vi "Begin.vi"(8 "error in":errorcluster) -> (0 "error out":errorcluster)   [LabVIEW 2014]
doc: "Called before other user functions, this VI is expected to open initial I/O refnums, load in file data, and do all program initialization. Notice that the <B>error out</B> terminal is simply used for data flow. Wiring it to other structures or subVIs ensures that this VI runs first."
uses:
  <vilib>/Rock Robotics/WPI/DriverStation/WPI_DriverStationRobotMode2.ctl
  <vilib>/Rock Robotics/WPI/Joystick/WPI_JoystickDeviceEnum.ctl
  <vilib>/Rock Robotics/SystemInterfaces/AI/FPGA_AIGyroChannel.ctl
  <vilib>/Rock Robotics/WPI/Camera/WPI_CameraWhite Balance Values.ctl
  <vilib>/Rock Robotics/WPI/Camera/WPI_CameraExposure Values.ctl
  <vilib>/Rock Robotics/WPI/Solenoid/WPI_SolenoidChannel.ctl
  <vilib>/Rock Robotics/SystemInterfaces/AI/FPGA_AIChannel.ctl
  <vilib>/Rock Robotics/WPI/Accelerometer/ADXL345 Range.ctl
  <vilib>/Rock Robotics/WPI/Accelerometer/WPI_AccelerometerADXL345 Axes.ctl
  <vilib>/Rock Robotics/SystemInterfaces/i2clib/i2c_bus.ctl
  <vilib>/Rock Robotics/SystemInterfaces/DIO/FPGA_DIOChannel.ctl
  <vilib>/Rock Robotics/SystemInterfaces/DIO/FPGA_DIOPWMChannel.ctl
  <vilib>/Rock Robotics/WPI/CAN/TalonSRX/WPI_CANTalonSRX_BrakeOverride.ctl
  Robot Global Data.vi
  <vilib>/Rock Robotics/WPI/RobotDrive/WPI_RobotDriveOpen4MotorWithCANJaguar.vi
  <vilib>/Rock Robotics/WPI/Solenoid/WPI_SolenoidOpenSingle.vi
  <vilib>/Rock Robotics/WPI/Counter/WPI_CounterDigitalInputToDigitalSource.vi
  <vilib>/Rock Robotics/WPI/MotorControl/WPI_MotorControlOpenCANTalonSRX.vi
  <vilib>/Rock Robotics/WPI/Compressor/WPI_CompressorGetSetRefNum.vi
panel:
  out "Discovered Devices":i32[](array[numeric])
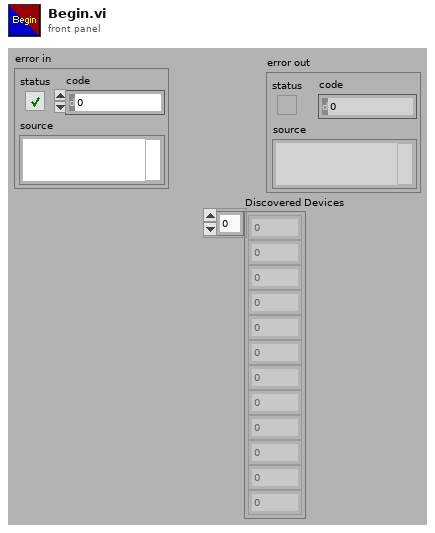
[diagram p1: front panel]
types:
  T1 = typedef "WPI_SolenoidChannel.ctl" = enum8{"Solenoid 0", "Solenoid 1", "Solenoid 2", "Solenoid 3", "Solenoid 4", "Solenoid 5", "Solenoid 6", "Solenoid 7", "Invalid"}
  T2 = typedef "WPI_CANTalonSRX_BrakeOverride.ctl" = enum8{"No Override", "Override to Coast", "Override to Brake"}
  T3 = typedef "FPGA_DIOChannel.ctl" = enum8{"DIO 0", "DIO 1", "DIO 2", "DIO 3", "DIO 4", "DIO 5", "DIO 6", "DIO 7", "DIO 8", "DIO 9", "DIO MXP 0", "DIO MXP 1", "DIO MXP 2", "DIO MXP 3", "DIO MXP 4", "DIO MXP 5", "DIO MXP 6", "DIO MXP 7", "DIO MXP 8", "DIO MXP 9", "DIO MXP 10", "DIO MXP 11", "DIO MXP 12", "DIO MXP 13", "DIO MXP 14", "DIO MXP 15", "Invalid"}
  T4 = typedef "FPGA_DIOPWMChannel.ctl" = enum8{"PWM 0", "PWM 1", "PWM 2", "PWM 3", "PWM 4", "PWM 5", "PWM 6", "PWM 7", "PWM 8", "PWM 9", "PWM MXP 0", "PWM MXP 1", "PWM MXP 2", "PWM MXP 3", "PWM MXP 4", "PWM MXP 5", "PWM MXP 6", "PWM MXP 7", "PWM MXP 8", "PWM MXP 9", "Invalid"}
  T5 = typedef "i2c_bus.ctl" = enum16{"I2C On-Board", "I2C MXP", "Invalid"}
  T6 = typedef "WPI_AccelerometerADXL345 Axes.ctl" = cluster{"X-Axis":bool, "Y-Axis":bool, "Z-Axis":bool}
  T7 = typedef "ADXL345 Range.ctl" = u8
  T8 = typedef "FPGA_AIChannel.ctl" = enum8{"AI 0", "AI 1", "AI 2", "AI 3", "AI MXP 0", "AI MXP 1", "AI MXP 2", "AI MXP 3", "Invalid"}
  T9 = typedef "WPI_CameraExposure Values.ctl" = enum16{"Auto", "Flicker-free 50 Hz", "Flicker-free 60 Hz", "Hold current", "Custom"}
  T10 = typedef "WPI_CameraWhite Balance Values.ctl" = enum16{"Auto", "Fixed indoor", "Fixed outdoor 1", "Fixed outdoor 2", "Fixed fluorescent 1", "Fixed fluorescent 2", "Hold current", "Custom"}
  T11 = typedef "FPGA_AIGyroChannel.ctl" = enum8{"AI 0", "AI 1", "Invalid"}
  T12 = typedef "WPI_JoystickDeviceEnum.ctl" = enum16{"USB 0", "USB 1", "USB 2", "USB 3", "USB 4", "USB 5"}
  T13 = typedef "WPI_DriverStationRobotMode2.ctl" = enum16{"Autonomous Disabled", "Autonomous Enabled", "Teleop Disabled", "Teleop Enabled", "Disconnected", "Finish", "Test Disabled", "Test Enabled", "Emergency Stopped"}
  T14 = typedef "WPI_JoystickDevRef.ctl" = cluster{"Device":T12}
  T15 = typedef "WPI_GyroDevRef.ctl" = cluster{"DevStatus":errorcluster, "Analog Module":T16, "Analog Channel":T8, "Offset":dbl, "Gain (VoltsPerDegree/Second)":dbl}
  T16 = typedef "FPGA_TypedefAnalogModule.ctl" = enum16{"Controller 1"}
  T17 = typedef "WPI_AccelerometerDevRef.ctl" = cluster{"DevStatus":errorcluster, "Controller":T16, "Scaling":T18, "Analog Channels":T19, "I2C Bus":T5, "SPI Bus":T20, "Accel Range":T7, "ADXL345 Axes":T6, "Handle":i32, "Device Address":u8, "Accel Type":enum16{"Analog", "ADXL345 I2C", "ADXL345 SPI", "Internal"}}
  T18 = typedef "WPI_AccelerometerScaling.ctl" = cluster{"Gain (VoltsPerG)":dbl, "Center Voltage":dbl}
  T19 = typedef "WPI_AccelerometerAnalogChannels.ctl" = cluster{"X-Axis":T8, "Y-Axis":T8, "Z-Axis":T8}
  T20 = typedef "spi_bus.ctl" = enum16{"SPI On-Board, CS0", "SPI On-Board, CS1", "SPI On-Board, CS2", "SPI On-Board, CS3", "SPI MXP", "Invalid"}
  T21 = typedef "WPI_RobotDriveDevRef.ctl" = cluster{"DevStatus":errorcluster, "Motors[]":T22[], "Square Inputs":bool, "Max Output":dbl}
  T22 = typedef "WPI_MotorControlDeviceRef.ctl" = cluster{"DeviceStatus":errorcluster, "Type":T23, "PWM":cluster{"Controller":T24, "PWM Channel":T4, "DeadBand":T25}, "CAN":cluster{"Device Number":u8, "Control Mode":T26, "Semaphore":T27, "Max Vout":dbl, "TalonSRX Control Mode":T28}, "Invert":bool, "TransformRef":T29, "InvTransformRef":T29}
  T23 = typedef "WPI_MotorControlType.ctl" = enum16{"PWM", "CAN", "CANTalonSRX"}
  T24 = typedef "FPGA_TypedefDigitalModule.ctl" = enum16{"Controller 1"}
  T25 = typedef "WPI_PWMDeadband.ctl" = cluster{"Name":string, "maxPositivePwm":i32, "minPositivePwm":i32, "centerPwm":i32, "maxNegativePwm":i32, "minNegativePwm":i32, "angularRange":u16}
  T26 = typedef "WPI_CANJaguar_ControlMode.ctl" = enum8{"Percent VBus", "Current", "Speed", "Position", "Voltage"}
  T27 = typedef "Semaphore RefNum" = refnum<k1>
  T28 = typedef "WPI_CANTalonSRX_APIControlMode.ctl" = enum8{"Percent VBus", "Speed", "Position", "Slave", "Unchanged / Invalid"}
  T29 = typedef "WPI_PWMTransform_ConPane.ctl" = refnum<vi>
  T30 = typedef "WPI_SolenoidDevRef.ctl" = cluster{"DevStatus":errorcluster, "Pneumatics Control Module":u8, "Forward Solenoid Channel":T1, "Reverse Solenoid Channel":T1}
  T31 = typedef "WPI_CameraDevRef.ctl" = cluster{"Camera Address":string, "CameraStatus":errorcluster}
  T32 = typedef "WPI_AnalogChannelDevRef.ctl" = cluster{"DevStatus":errorcluster, "Controller":T16, "Analog Channel":T8}
  T33 = typedef "WPI_I2CDevRef.ctl" = cluster{"DevStatus":errorcluster, "Controller":T24, "Device Address":u8, "Handle":i32, "I2C Bus":T5}
  T34 = typedef "WPI_CompressorDevRef.ctl" = cluster{"DevStatus":errorcluster, "Pneumatics Control Module":u8}
  T35 = typedef "WPI_DigitalInputDevRef.ctl" = cluster{"DevStatus":errorcluster, "DIO Channel":T3, "Controller":T24}
  T36 = typedef "WPI_ServoDeviceRef.ctl" = cluster{"DeviceStatus":errorcluster, "Controller":T24, "PWM Channel":T4, "DeadBand":T25}
  T37 = typedef "FPGA_CounterEncoderSourceConvertionLVSourceType.ctl" = cluster{"DevStatus":errorcluster, "AnalogTriggerMode?":bool, "DigitalMode":cluster{"Controller":T24, "DIO Channel":T38}, "AnalogTriggerMode":cluster{"AnalogTriggerIndex":T39, "OutputType":T40}}
  T38 = typedef "FPGA_DIODigitalSourceChannel.ctl" = enum8{"DIO 0", "DIO 1", "DIO 2", "DIO 3", "DIO 4", "DIO 5", "DIO 6", "DIO 7", "DIO 8", "DIO 9", "DIO MXP 0", "DIO MXP 1", "DIO MXP 2", "DIO MXP 3", "DIO MXP 4", "DIO MXP 5", "DIO MXP 6", "DIO MXP 7", "DIO MXP 8", "DIO MXP 9", "DIO MXP 10", "DIO MXP 11", "DIO MXP 12", "DIO MXP 13", "DIO MXP 14", "DIO MXP 15", "Disabled"}
  T39 = typedef "FPGA_AnalogTriggerIndex.ctl" = enum8{"Trig 0", "Trig 1", "Trig 2", "Trig 3", "Trig 4", "Trig 5", "Trig 6", "Trig 7", "Invalid"}
  T40 = typedef "FPGA_AnalogTriggerOutType.ctl" = enum16{"InWindow", "TriggerState", "Rising", "Falling"}
  T41 = typedef "WPI_EncoderDevRef.ctl" = cluster{"DevStatus":errorcluster, "EncoderIndex":T42, "CounterIndex":T43, "DistancePerCount":dbl, "Decoding Type":T44}
  T42 = typedef "FPGA_EncoderIdx.ctl" = enum8{"Enc 0", "Enc 1", "Enc 2", "Enc 3", "Enc 4", "Enc 5", "Enc 6", "Enc 7", "Invalid"}
  T43 = typedef "FPGA_CounterCtrSystemIndex.ctl" = enum8{"Ctr 0", "Ctr 1", "Ctr 2", "Ctr 3", "Ctr 4", "Ctr 5", "Ctr 6", "Ctr 7", "Invalid"}
  T44 = typedef "WPI_EncoderType.ctl" = enum16{"1x", "2x", "4x"}
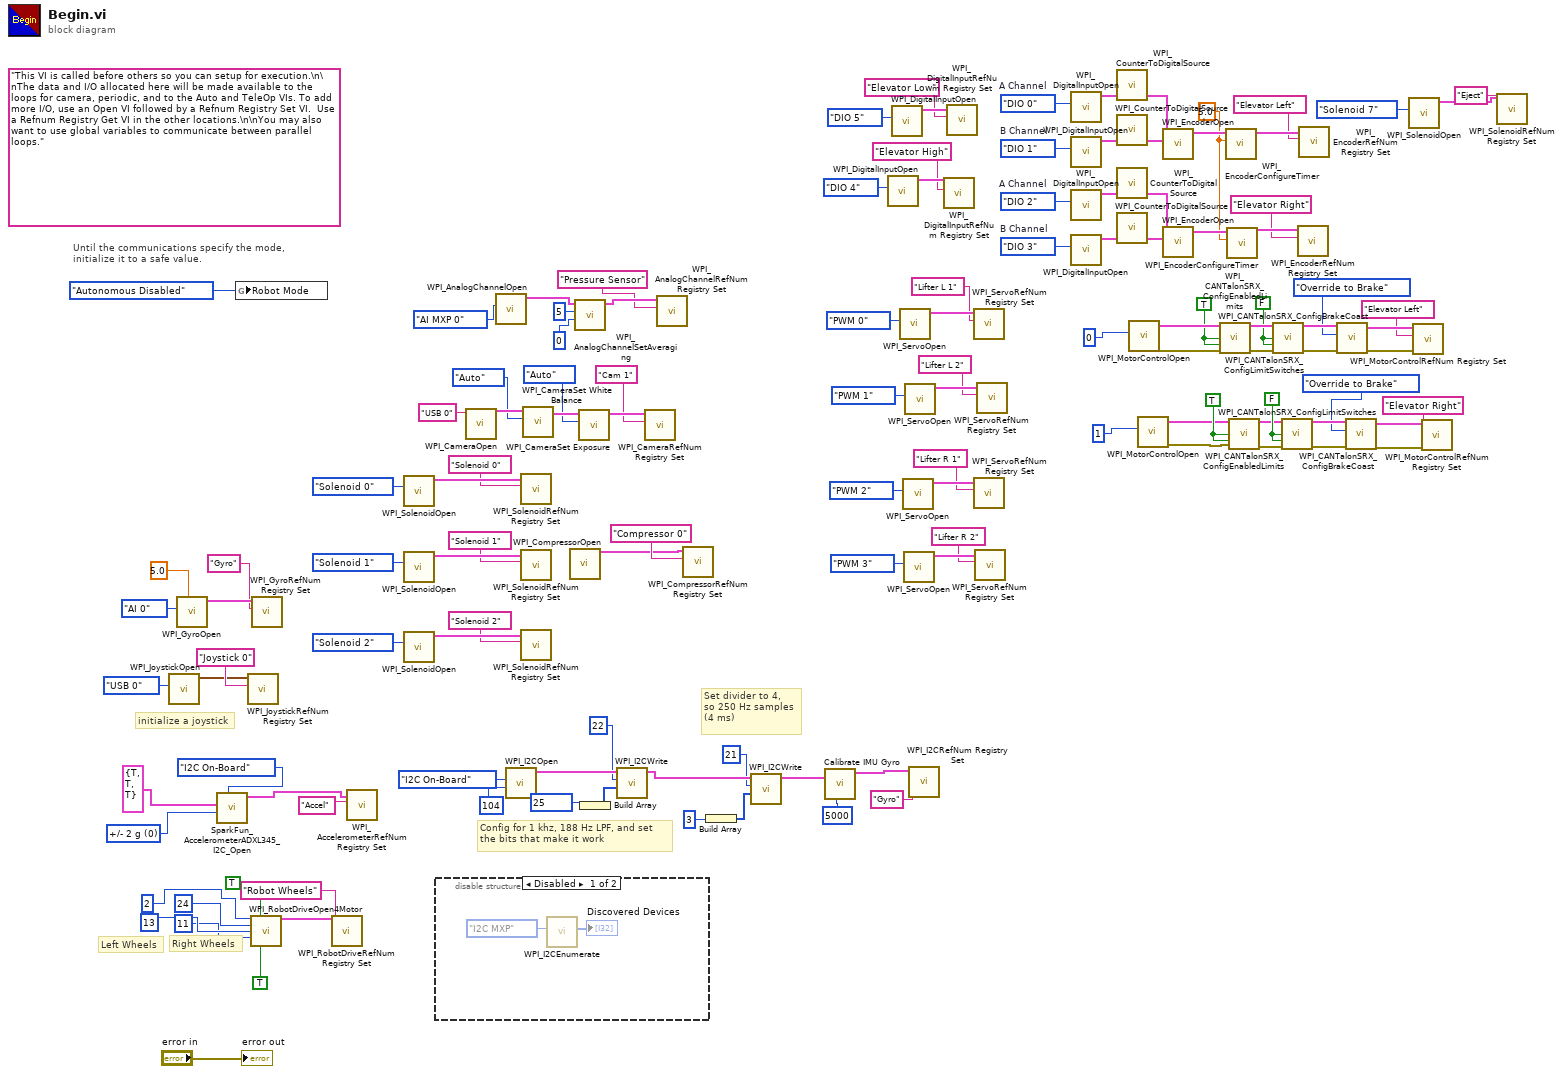
[diagram p0: block diagram]
diagram:
  w17 = FALSE ("Forward Limit Switch Enable")
  w15 = TRUE ("Forward Limit Switch Enable")
  w25 = FALSE ("Forward Limit Switch Enable")
  w27 = TRUE ("Forward Limit Switch Enable")
  w30 = 5.0 ("Minimum Rate")
  w55 = FPGA_DIOChannel."DIO 3"  # B Channel
  w56 = FPGA_DIOChannel."DIO 2"  # A Channel
  w66 = FPGA_DIOChannel."DIO 1"  # B Channel
  w65 = FPGA_DIOChannel."DIO 0"  # A Channel
  w82 = T7 0 items=["+/- 2 g", "+/- 4 g", "+/- 8 g", "+/- 16 g"] ("Accel Range")
  (unwired) "This VI is called before others so you can setup for execution.\n\nThe data and I/O allocated here will be made available to the loops for camera, periodic, and to the Auto and TeleOp VIs. To add more I/O, use an Open VI followed by a Refnum Registry Set VI.  Use a Refnum Registry Get VI in the other locations.\n\nYou may also want to use global variables to communicate between parallel loops."
  # "Set divider to 4, \nso 250 Hz samples\n(4 ms)"
  # "Config for 1 khz, 188 Hz LPF, and set\nthe bits that make it work"
  # "Right Wheels"
  # "Left Wheels"
  # "initialize a joystick"
  # "Until the communications specify the mode,\ninitialize it to a safe value."
  n1 = call <vilib>:"WPI_JoystickOpen.vi"("JoystickDevice"=WPI_JoystickDeviceEnum."USB 0") -> ("JoystickDevRef"=w124:T14)  [unwired: 10 in]
  n2 = call <vilib>:"WPI_GyroOpen.vi"("Calibration Time (s)"=5.0, "Analog Channel"=FPGA_AIGyroChannel."AI 0") -> ("GyroDevRef"=w115:T15)  [unwired: 7 in, 2 out]
  n3 = call "SparkFun_AccelerometerADXL345_I2C_Open.vi"("I2C Bus"=i2c_bus."I2C On-Board", "Accel Range"=w82, "ADXL345 Axes"=T6 {"X-Axis"=TRUE, "Y-Axis"=TRUE, "Z-Axis"=TRUE}) -> ("AccelerometerDevRef"=w84:T17)  [unwired: 7 in, 1 out]
  n4 = global write "Robot Global Data.vi" "Robot Mode"(WPI_DriverStationRobotMode2."Autonomous Disabled" ("Robot Mode")) -> ()
  n5 = call <vilib>:"WPI_JoystickRefNum Registry Set.vi"("refnum name"="Joystick 0", "JoystickDevRef"=w124) -> ()  [unwired: 8 in, 2 out]
  n6 = call-poly <vilib>:"WPI_RobotDriveOpen4Motor.vi"("Rear Left Motor"=u8 2, "Rear Left Motor Inverted"=TRUE, "Rear Right Motor"=u8 24, "Front Left Motor"=u8 13, "Front Right Motor"=u8 11, "Front Left Motor Inverted"=TRUE) -> ("RobotDriveDevRef"=w121:T21)  [unwired: 8 in, 1 out]
  n7 = call <vilib>:"WPI_GyroRefNum Registry Set.vi"("refnum name"="Gyro", "GyroDevRef"=w115) -> ()  [unwired: 8 in, 2 out]
  n8 = call <vilib>:"WPI_RobotDriveRefNum Registry Set.vi"("refnum name"="Robot Wheels", "RobotDriveDevRef"=w121) -> ()  [unwired: 8 in, 2 out]
  n9 = call <vilib>:"WPI_AccelerometerRefNum Registry Set.vi"("refnum name"="Accel", "AccelerometerDevRef"=w84) -> ()  [unwired: 8 in, 2 out]
  n10 = call-poly <vilib>:"WPI_SolenoidOpen.vi"("Solenoid Channel"=WPI_SolenoidChannel."Solenoid 0") -> ("SolenoidDevRef"=w102:T30)  [unwired: 9 in, 1 out]
  n11 = call-poly <vilib>:"WPI_SolenoidOpen.vi"("Solenoid Channel"=WPI_SolenoidChannel."Solenoid 1") -> ("SolenoidDevRef"=w94:T30)  [unwired: 9 in, 1 out]
  n12 = call-poly <vilib>:"WPI_SolenoidOpen.vi"("Solenoid Channel"=WPI_SolenoidChannel."Solenoid 2") -> ("SolenoidDevRef"=w97:T30)  [unwired: 9 in, 1 out]
  n13 = disable-structure shown="Disabled" {
    frame Disabled {
      n14 = call <vilib>:"WPI_I2CEnumerate.vi"("I2C Bus"=i2c_bus."I2C MXP") -> ("Discovered Devices"=→"Discovered Devices":i32[])  [unwired: 10 in]
    }
    frame Enabled {
    }
  }
  n15 = call <vilib>:"WPI_CameraOpen.vi"("Camera Address"="USB 0") -> ("CameraDevRef"=w108:T31)  [unwired: 9 in, 1 out]
  n16 = call <vilib>:"WPI_AnalogChannelOpen.vi"("Analog Channel"=FPGA_AIChannel."AI MXP 0") -> ("AIDeviceRef"=w90:T32)  [unwired: 9 in, 1 out]
  n17 = call <vilib>:"WPI_I2COpen.vi"("Device Address"=104, "I2C Bus"=i2c_bus."I2C On-Board") -> ("I2CDevRef"=w75:T33)  [unwired: 8 in, 1 out]
  n18 = call <vilib>:"WPI_SolenoidRefNum Registry Set.vi"("refnum name"="Solenoid 0", "SolenoidDevRef"=w102) -> ()  [unwired: 8 in, 2 out]
  n19 = call <vilib>:"WPI_SolenoidRefNum Registry Set.vi"("refnum name"="Solenoid 1", "SolenoidDevRef"=w94) -> ()  [unwired: 8 in, 2 out]
  n20 = call <vilib>:"WPI_SolenoidRefNum Registry Set.vi"("refnum name"="Solenoid 2", "SolenoidDevRef"=w97) -> ()  [unwired: 8 in, 2 out]
  n21 = call <vilib>:"WPI_CameraSet White Balance.vi"("White Balance"=WPI_CameraWhite_Balance_Values."Auto", "CameraDevRef"=w108) -> ("CameraDevRef Out"=w106:T31)  [unwired: 8 in, 1 out]
  n22 = call <vilib>:"WPI_CompressorOpen.vi"() -> ("CompressorDevRef"=w98:T34)  [unwired: 14 in, 1 out]
  n23 = call <vilib>:"WPI_AnalogChannelSetAveraging.vi"("OversampleBits"=u8 0, "AverageBits"=u8 5, "AIDeviceRef"=w90) -> ("AIDeviceRef"=w91:T32)  [unwired: 7 in, 1 out]
  n24 = call <vilib>:"WPI_CameraSet Exposure.vi"("Exposure"=WPI_CameraExposure_Values."Auto", "CameraDevRef"=w106) -> ("CameraDevRef Out"=w104:T31)  [unwired: 8 in, 1 out]
  n25 = Build Array(u8 25) -> (w77:u8[])
  n26 = call <vilib>:"WPI_I2CWrite.vi"("I2CDataToSend"=w77, "I2CRegister"=u8 22, "I2CDevRef"=w75) -> ("I2CDevRef"=w78:T33)  [unwired: 7 in, 1 out]
  n27 = call <vilib>:"WPI_CameraRefNum Registry Set.vi"("refnum name"="Cam 1", "CameraDevRef"=w104) -> ()  [unwired: 8 in, 2 out]
  n28 = call <vilib>:"WPI_AnalogChannelRefNum Registry Set.vi"("refnum name"="Pressure Sensor", "AIDeviceRef"=w91) -> ()  [unwired: 8 in, 2 out]
  n29 = call <vilib>:"WPI_CompressorRefNum Registry Set.vi"("refnum name"="Compressor 0", "CompressorDevRef"=w98) -> ()  [unwired: 8 in, 2 out]
  n30 = Build Array(u8 3) -> (w72:u8[])
  n31 = call <vilib>:"WPI_I2CWrite.vi"("I2CDataToSend"=w72, "I2CRegister"=u8 21, "I2CDevRef"=w78) -> ("I2CDevRef"=w79:T33)  [unwired: 7 in, 1 out]
  n32 = call "Calibrate IMU Gyro.vi"("Calib time (ms)"=u32 5000, "I2CDevRef in"=w79) -> ("I2CDevRef out"=w80:T33)  [unwired: 9 in]
  n33 = call <vilib>:"WPI_DigitalInputOpen.vi"("DIO Channel"=FPGA_DIOChannel."DIO 4") -> ("DigitalInputDevRef"=w47:T35)  [unwired: 9 in, 1 out]
  n34 = call <vilib>:"WPI_DigitalInputOpen.vi"("DIO Channel"=FPGA_DIOChannel."DIO 5") -> ("DigitalInputDevRef"=w48:T35)  [unwired: 9 in, 1 out]
  n35 = call <vilib>:"WPI_ServoOpen.vi"("PWM Channel"=FPGA_DIOPWMChannel."PWM 0") -> ("ServoDeviceRef"=w38:T36)  [unwired: 9 in, 1 out]
  n36 = call <vilib>:"WPI_ServoOpen.vi"("PWM Channel"=FPGA_DIOPWMChannel."PWM 2") -> ("ServoDeviceRef"=w36:T36)  [unwired: 9 in, 1 out]
  n37 = call <vilib>:"WPI_ServoOpen.vi"("PWM Channel"=FPGA_DIOPWMChannel."PWM 3") -> ("ServoDeviceRef"=w35:T36)  [unwired: 9 in, 1 out]
  n38 = call <vilib>:"WPI_ServoOpen.vi"("PWM Channel"=FPGA_DIOPWMChannel."PWM 1") -> ("ServoDeviceRef"=w37:T36)  [unwired: 9 in, 1 out]
  n39 = call <vilib>:"WPI_I2CRefNum Registry Set.vi"("refnum name"="Gyro", "I2CDevRef"=w80) -> ()  [unwired: 8 in, 2 out]
  n40 = call <vilib>:"WPI_DigitalInputRefNum Registry Set.vi"("refnum name"="Elevator High", "DigitalInputDevRef"=w47) -> ()  [unwired: 8 in, 2 out]
  n41 = call <vilib>:"WPI_DigitalInputRefNum Registry Set.vi"("refnum name"="Elevator Low", "DigitalInputDevRef"=w48) -> ()  [unwired: 8 in, 2 out]
  n42 = call <vilib>:"WPI_ServoRefNum Registry Set.vi"("refnum name"="Lifter L 1", "ServoDeviceRef"=w38) -> ()  [unwired: 8 in, 2 out]
  n43 = call <vilib>:"WPI_ServoRefNum Registry Set.vi"("refnum name"="Lifter R 1", "ServoDeviceRef"=w36) -> ()  [unwired: 8 in, 2 out]
  n44 = call <vilib>:"WPI_ServoRefNum Registry Set.vi"("refnum name"="Lifter R 2", "ServoDeviceRef"=w35) -> ()  [unwired: 8 in, 2 out]
  n45 = call <vilib>:"WPI_ServoRefNum Registry Set.vi"("refnum name"="Lifter L 2", "ServoDeviceRef"=w37) -> ()  [unwired: 8 in, 2 out]
  n46 = call <vilib>:"WPI_DigitalInputOpen.vi"("DIO Channel"=w65) -> ("DigitalInputDevRef"=w62:T35)  [unwired: 2 in, 8 out]
  n47 = call <vilib>:"WPI_DigitalInputOpen.vi"("DIO Channel"=w66) -> ("DigitalInputDevRef"=w63:T35)  [unwired: 2 in, 8 out]
  n48 = call <vilib>:"WPI_DigitalInputOpen.vi"("DIO Channel"=w56) -> ("DigitalInputDevRef"=w59:T35)  [unwired: 2 in, 8 out]
  n49 = call <vilib>:"WPI_DigitalInputOpen.vi"("DIO Channel"=w55) -> ("DigitalInputDevRef"=w58:T35)  [unwired: 2 in, 8 out]
  n50 = call-poly <vilib>:"WPI_CounterToDigitalSource.vi"("DigitalInputDevRef"=w62) -> ("Digital Source"=w61:T37)  [unwired: 6 out]
  n51 = call-poly <vilib>:"WPI_CounterToDigitalSource.vi"("DigitalInputDevRef"=w63) -> ("Digital Source"=w64:T37)  [unwired: 6 out]
  n52 = call-poly <vilib>:"WPI_CounterToDigitalSource.vi"("DigitalInputDevRef"=w59) -> ("Digital Source"=w60:T37)  [unwired: 6 out]
  n53 = call-poly <vilib>:"WPI_CounterToDigitalSource.vi"("DigitalInputDevRef"=w58) -> ("Digital Source"=w57:T37)  [unwired: 6 out]
  n54 = call-poly <vilib>:"WPI_MotorControlOpen.vi"("Device Number"=u8 0) -> ("error out"=w9:errorcluster, "MotorControlDeviceRef"=w28:T22)  [unwired: 9 in]
  n55 = call-poly <vilib>:"WPI_MotorControlOpen.vi"("Device Number"=u8 1) -> ("error out"=w8:errorcluster, "MotorControlDeviceRef"=w14:T22)  [unwired: 9 in]
  n56 = call <vilib>:"WPI_EncoderOpen.vi"("BSource"=w64, "ASource"=w61) -> ("EncoderDevRef"=w44:T41)  [unwired: 6 in, 3 out]
  n57 = call <vilib>:"WPI_EncoderOpen.vi"("BSource"=w57, "ASource"=w60) -> ("EncoderDevRef"=w43:T41)  [unwired: 6 in, 3 out]
  n58 = call <vilib>:"WPI_CANTalonSRX_ConfigEnabledLimits.vi"("CAN Talon SRX Ref"=w28, "Forward Limit Switch Enable"=w27, "Reverse Limit Switch Enable"=w27, "error in (no error)"=w9) -> ("CAN Talon SRX Ref Out"=w26:T22, "error out"=w11:errorcluster)  [unwired: 10 in]
  n59 = call <vilib>:"WPI_EncoderConfigureTimer.vi"("Minimum Rate"=w30, "EncoderDevRef"=w44) -> ("EncoderDevRef"=w41:T41)  [unwired: 8 in, 1 out]
  n60 = call <vilib>:"WPI_EncoderConfigureTimer.vi"("Minimum Rate"=w30, "EncoderDevRef"=w43) -> ("EncoderDevRef"=w42:T41)  [unwired: 8 in, 1 out]
  n61 = call <vilib>:"WPI_CANTalonSRX_ConfigEnabledLimits.vi"("CAN Talon SRX Ref"=w14, "Forward Limit Switch Enable"=w15, "Reverse Limit Switch Enable"=w15, "error in (no error)"=w8) -> ("CAN Talon SRX Ref Out"=w16:T22, "error out"=w10:errorcluster)  [unwired: 10 in]
  n62 = call <vilib>:"WPI_CANTalonSRX_ConfigLimitSwitches.vi"("CAN Talon SRX Ref"=w26, "Forward Limit Switch Normally Open"=w25, "Reverse Limit Switch Normally Open"=w25, "error in (no error)"=w11) -> ("CAN Talon SRX Ref Out"=w24:T22, "error out"=w7:errorcluster)  [unwired: 10 in]
  n63 = call <vilib>:"WPI_CANTalonSRX_ConfigLimitSwitches.vi"("CAN Talon SRX Ref"=w16, "Forward Limit Switch Normally Open"=w17, "Reverse Limit Switch Normally Open"=w17, "error in (no error)"=w10) -> ("CAN Talon SRX Ref Out"=w18:T22, "error out"=w4:errorcluster)  [unwired: 10 in]
  n64 = call <vilib>:"WPI_EncoderRefNum Registry Set.vi"("refnum name"="Elevator Right", "EncoderDevRef"=w42) -> ()  [unwired: 8 in, 2 out]
  n65 = call <vilib>:"WPI_EncoderRefNum Registry Set.vi"("refnum name"="Elevator Left", "EncoderDevRef"=w41) -> ()  [unwired: 8 in, 2 out]
  n66 = call <vilib>:"WPI_CANTalonSRX_ConfigBrakeCoast.vi"("error in (no error)"=w7, "Brake / Coast Mode"=WPI_CANTalonSRX_BrakeOverride."Override to Brake", "CAN Talon SRX Ref"=w24) -> ("error out"=w6:errorcluster, "CAN Talon SRX Ref Out"=w22:T22)  [unwired: 7 in]
  n67 = call <vilib>:"WPI_CANTalonSRX_ConfigBrakeCoast.vi"("error in (no error)"=w4, "Brake / Coast Mode"=WPI_CANTalonSRX_BrakeOverride."Override to Brake", "CAN Talon SRX Ref"=w18) -> ("error out"=w5:errorcluster, "CAN Talon SRX Ref Out"=w19:T22)  [unwired: 7 in]
  n68 = call-poly <vilib>:"WPI_SolenoidOpen.vi"("Solenoid Channel"=WPI_SolenoidChannel."Solenoid 7") -> ("SolenoidDevRef"=w2:T30)  [unwired: 9 in, 1 out]
  n69 = call <vilib>:"WPI_MotorControlRefNum Registry Set.vi"("error in (no error)"=w6, "refnum name"="Elevator Left", "MotorControlDevRef"=w22) -> ()  [unwired: 7 in, 2 out]
  n70 = call <vilib>:"WPI_MotorControlRefNum Registry Set.vi"("error in (no error)"=w5, "refnum name"="Elevator Right", "MotorControlDevRef"=w19) -> ()  [unwired: 7 in, 2 out]
  n71 = call <vilib>:"WPI_SolenoidRefNum Registry Set.vi"("refnum name"="Eject", "SolenoidDevRef"=w2) -> ()  [unwired: 8 in, 2 out]
  "error out" <- "error in"
